vi "GetGP275Pressure.vi"() -> (3 "Pressure (Torr)":sgl)   [LabVIEW 2011]
uses:
  GlobalVariables.vi
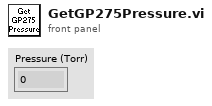
[diagram p1: front panel]
types:
  T1 = typedef "GP275 Cluster.ctl" = cluster{"Pressure (Torr)":sgl}
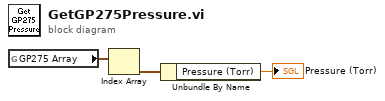
[diagram p0: block diagram]
diagram:
  n1 = global read "GlobalVariables.vi" "GP275 Array"() -> (w3:T1[])
  n2 = Index Array(array=w3) -> (element=w2:T1)  [unwired: 1 in]
  n3 = Unbundle By Name(w2) -> ("Pressure (Torr)"=→"Pressure (Torr)":sgl)
